vi "MT Generate FSK System Parameters(map).vi"(0 "samples per symbol (16)":i32=16, 5 "symbol values":i32[](array[numeric]), 7 "FSK deviation (Hz)":dbl=150000.0 format="%.2p", 9 "symbol phase continuity":enum16{"continuous", "discontinuous"}(ring), 11 "error in (no error)":errorcluster) -> (6 "FSK system parameters":T1 {"symbol map" format="%.2f"}, 8 "bits per symbol":i32, 15 "error out":errorcluster)   [LabVIEW 2020, in "niDMT.lvlib"]
doc: "This polymorphic instance calculates parameters for use with either the MT Modulate FSK or MT Demodulate FSK VI. This VI accepts an input array of <B>symbol values</B> that explicitly specifies the positions of the symbol map."
uses:
  <vilib>/addons/Modulation/niDMT.lvlib
  <vilib>/addons/Modulation/Digital/Support/Controls/FSK System Parameters.ctl
  <vilib>/Analysis/1siggen.llb/Ramp Pattern by Samples.vi
  <vilib>/addons/Modulation/niAMT.lvlib
  <vilib>/Analysis/NI_AALBase.lvlib
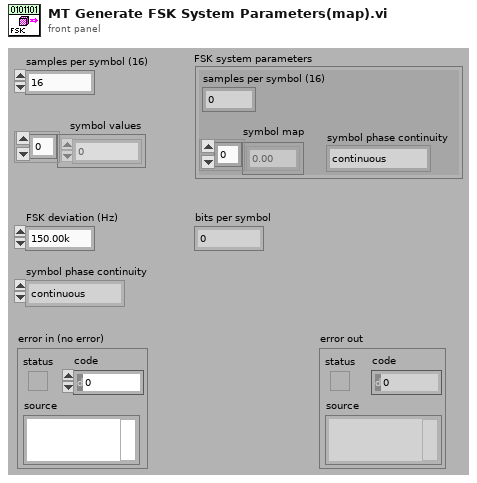
[diagram p1: front panel]
types:
  T1 = cluster{"samples per symbol (16)":i32, "symbol map":dbl[], "symbol phase continuity":enum16{"continuous", "discontinuous"}}
  T2 = typedef "niDMT.lvlib/FSK System Parameters.ctl" = cluster{"samples per symbol (16)":i32, "symbol map":dbl[], "symbol phase continuity":enum16{"continuous", "discontinuous"}}
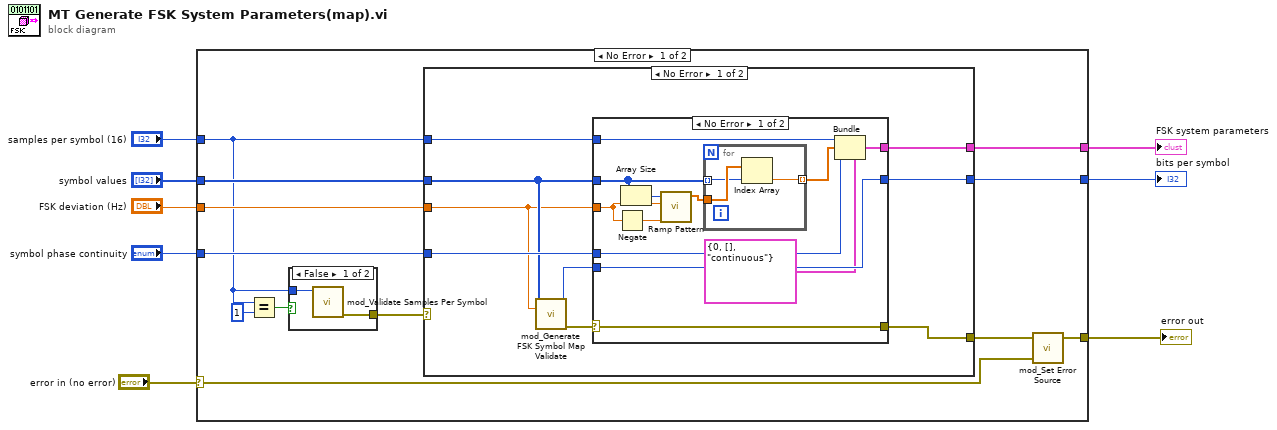
[diagram p0: block diagram]
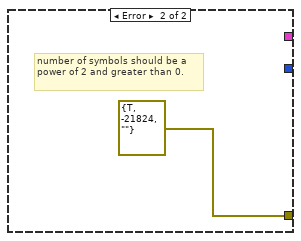
[diagram p3: hidden frame]
diagram:
  n1 = case shown="No Error" "error in (no error)" {
    selector: "error in (no error)" -> [w15 w49]
    tunnel: "samples per symbol (16)" -> [w11 _]
    tunnel: "symbol phase continuity" -> [w20 _]
    tunnel: "symbol values" -> [w13 _]
    tunnel: [w19 _] -> w5
    tunnel: "FSK deviation (Hz)" -> [w18 _]
    tunnel: [w17 _] -> w3
    tunnel: [w16 w49] -> w1
    frame No Error {
      n2 = Equal?(x=w11, y=1) -> (x = y?=w9:bool)
      n3 = case shown="False" w9 {
        tunnel: w11 -> [w22 _]
        tunnel: [w21 _] -> w12
        frame False {
          n4 = call <vilib>:"mod_Validate Samples Per Symbol.vi"("Samples Per Symbol"=w22) -> ("error out"=w21:errorcluster)  [unwired: 10 out]
        }
        frame True {
        }
      }
      n5 = case shown="No Error" w12 {
        selector: w12 -> [_ w48]
        tunnel: w11 -> [w31 _]
        tunnel: w20 -> [w30 _]
        tunnel: [w29 _] -> w19
        tunnel: w18 -> [w23 _]
        tunnel: [w28 _] -> w17
        tunnel: [w27 w48] -> w14
        tunnel: w13 -> [w24 _]
        frame No Error {
          n6 = call <vilib>:"mod_Generate FSK Symbol Map Validate.vi"("Symbol Map"=w24, "deviation"=w23) -> ("bits per symbol"=w25:i32, "error out"=w26:errorcluster)  [unwired: 12 out]
          n7 = case shown="No Error" w26 {
            selector: w26 -> [w37 _]
            tunnel: w31 -> [w43 _]
            tunnel: w30 -> [w41 _]
            tunnel: w24 -> [w34 _]
            tunnel: [w40 _] -> w29
            tunnel: w23 -> [w39 _]
            tunnel: [w38 _] -> w28
            tunnel: w25 -> [w38 _]
            tunnel: [w37 errorcluster {"status"=TRUE, "code"=-21824, "source"=""} ("final error in (no error)")] -> w27
            frame No Error {
              n8 = Negate(x=w39) -> (-x=w42:dbl)
              n9 = Array Size(array=w34) -> (size(s)=w36:i32)
              n10 = call-poly <vilib>:"Ramp Pattern.vi"("start"=w42, "end"=w39, "samples"=w36) -> ("Ramp Pattern"=w35:dbl[])  [unwired: 7 in, 1 out]
              n11 = for {
                tunnel: w35 -> [w46]
                tunnel: w34 -> [w45] mode=indexing
                tunnel: [w44] -> w33 mode=indexing
                n12 = Index Array(array=w46, index=w45) -> (element=w44:dbl)
              }
              n13 = Bundle(cluster=T2 {"samples per symbol (16)"=0, "symbol map"=[], "symbol phase continuity"=enum."continuous"} ("FSK system parameters"), "samples per symbol (16)"=w43, "symbol map"=w33, "symbol phase continuity"=w41) -> (w40:T2)
            }
            frame Error {
              # "number of symbols should be a power of 2 and greater than 0."
            }
          }
        }
        frame Error {
        }
      }
      n14 = call <vilib>:"mod_Set Error Source.vi"("initial error in (no error)"=w15, "final error in (no error)"=w14) -> ("error out"=w16:errorcluster)  [unwired: 3 out]
    }
    frame Error {
    }
  }
  "FSK system parameters" <- w5
  "bits per symbol" <- w3
  "error out" <- w1
